vi "Smart IO Functions.vi"() -> ()   [LabVIEW 2026]
uses:
  MrcLib.lvlib
panel:
  out "Raw Value":u32
  out "Voltage":dbl
  out "error out":errorcluster
  in  "buffer Data":u32[](array[colorbox])=[1250047, 8191, 16718848, 16732482]
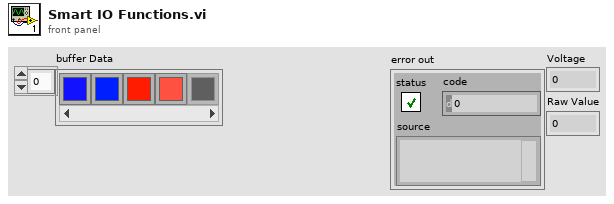
[diagram p1: front panel]
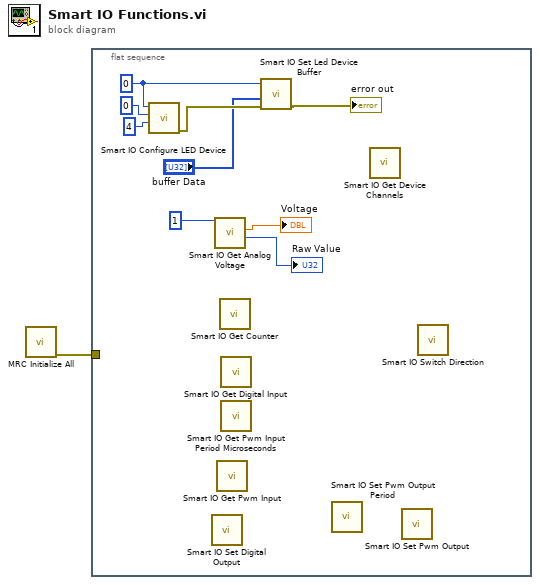
[diagram p0: block diagram]
diagram:
  n1 = call "MRC Initialize All.vi"() -> ("error out"=w1:errorcluster)  [unwired: 11 in]
  n2 = flat-sequence {
    tunnel: w1 -> [_]
    frame #0 {
      w8 = 0 ("deviceIndex")
      n3 = call "Smart IO Configure LED Device.vi"("length"=4, "startIndex"=0, "deviceIndex"=w8) -> ("error out"=w10:errorcluster)  [unwired: 7 in, 1 out]
      n4 = call "Smart IO Set Digital Output.vi"() -> ()  [unwired: 11 in, 1 out]
      n5 = call "Smart IO Get Analog Voltage.vi"("deviceIndex"=1) -> ("Raw Value"=→"Raw Value":u32, "Voltage"=→"Voltage":dbl)  [unwired: 8 in, 1 out]
      n6 = call "Smart IO Get Pwm Input.vi"() -> ()  [unwired: 9 in, 3 out]
      n7 = call "Smart IO Get Counter.vi"() -> ()  [unwired: 10 in, 2 out]
      n8 = call "Smart IO Get Digital Input.vi"() -> ()  [unwired: 10 in, 2 out]
      n9 = call "Smart IO Get Pwm Input Period Microseconds.vi"() -> ()  [unwired: 10 in, 2 out]
      n10 = call "Smart IO Set Led Device Buffer.vi"("error in (no error)"=w10, "buffer Data"="buffer Data", "deviceIndex"=w8) -> ("error out"=→"error out":errorcluster)  [unwired: 8 in]
      n11 = call "Smart IO Set Pwm Output Period.vi"() -> ()  [unwired: 11 in, 1 out]
      n12 = call "Smart IO Get Device Channels.vi"() -> ()  [unwired: 10 in, 2 out]
      n13 = call "Smart IO Set Pwm Output.vi"() -> ()  [unwired: 11 in, 1 out]
      n14 = call "Smart IO Switch Direction.vi"() -> ()  [unwired: 11 in, 1 out]
    }
  }
